vi "ziSaveSettings.vi"(3 "Error In":errorcluster, 4 "Path (\"\")":string, 5 "file path (dialog if empty)":path, 6 "Handle In":T1 {"Handle" format="0x%08x"; "Conn" format="0x%08x"}) -> (0 "Error Out":errorcluster, 1 "Saved Array":string[][](array[string]), 2 "Handle Out":T1 {"Handle" format="0x%08x"; "Conn" format="0x%08x"})   [LabVIEW 2015, in "Zurich Instruments LabOne.lvlib"]
uses:
  Zurich Instruments LabOne.lvlib
  <vilib>/Utility/file.llb/Write To Spreadsheet File (string).vi
  <vilib>/regexp/Match Regular Expression.xnode
  ziTypeHandle.ctl
panel:
  out "node_paths":string[](array[string])
  out "node_values":string[](array[string])
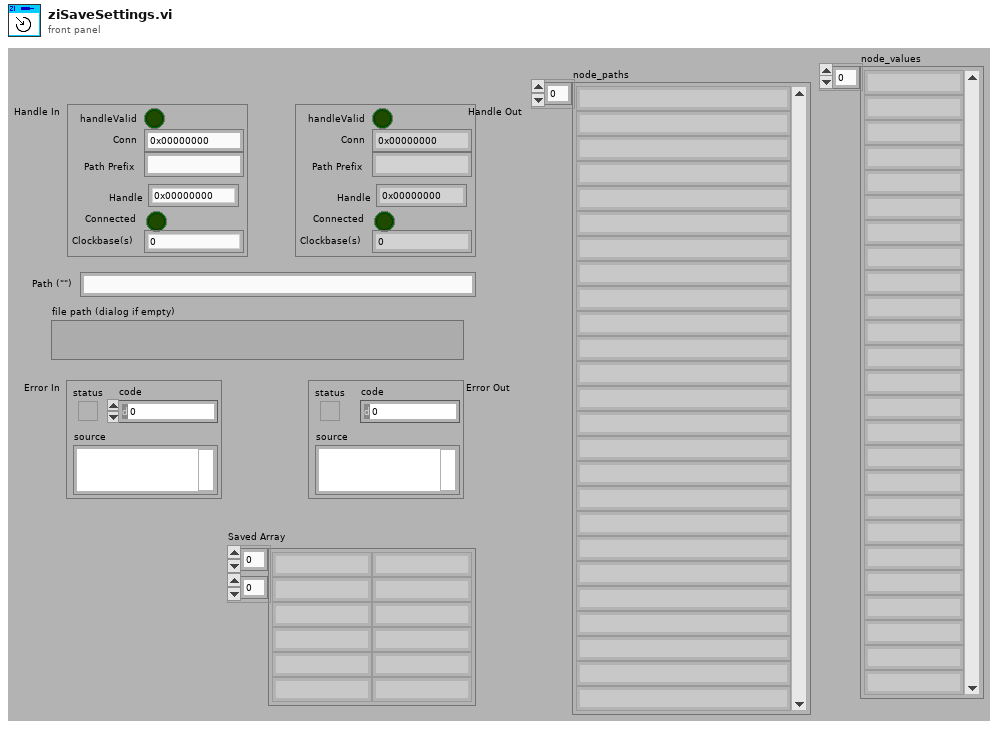
[diagram p1: front panel]
types:
  T1 = typedef "Zurich Instruments LabOne.lvlib/ziTypeHandle.ctl" = cluster{"handleValid":bool, "Conn":u64, "Path Prefix":string, "Handle":u64, "Connected":bool, "Clockbase(s)":dbl}
  T2 = cluster{"Recursive":bool, "Absolut":bool, "Leafs Only":bool, "Settings Only":bool}
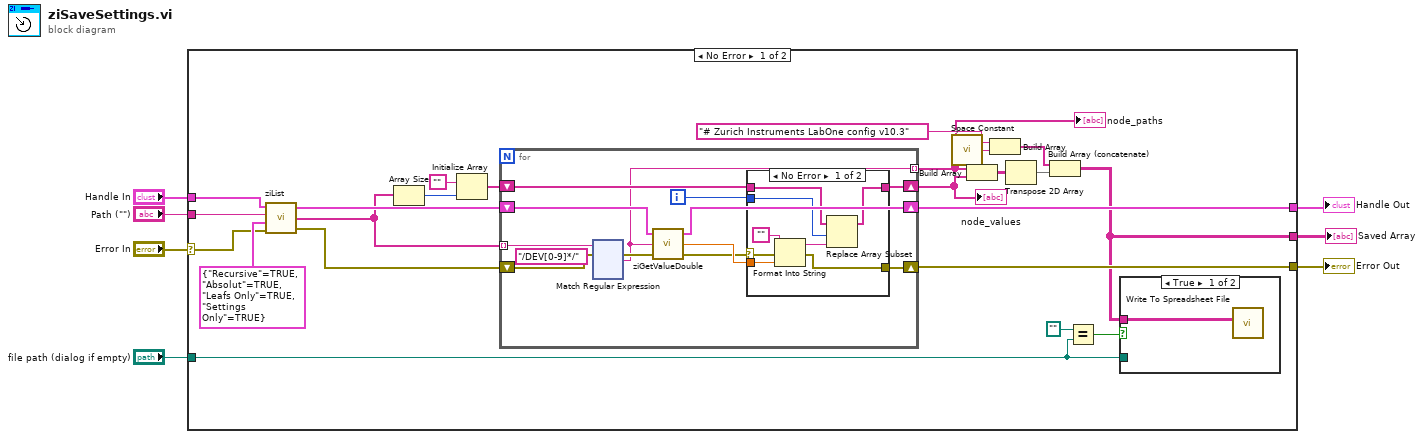
[diagram p0: block diagram]
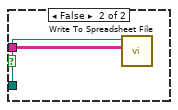
[diagram p2: hidden frame]
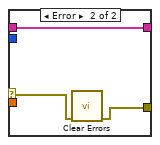
[diagram p3: hidden frame]
diagram:
  n1 = case shown="No Error" "Error In" {
    selector: "Error In" -> [w8 w164]
    tunnel: [w28 w165] -> w7
    tunnel: [w27 w164] -> w6
    tunnel: "file path (dialog if empty)" -> [w11 _]
    tunnel: "Handle In" -> [w25 w165]
    tunnel: "Path (\"\")" -> [w24 _]
    tunnel: [w15 _] -> w2
    frame No Error {
      n2 = call "ziList.vi"("Error In"=w8, "Flags (None)"=T2 {"Recursive"=TRUE, "Absolut"=TRUE, "Leafs Only"=TRUE, "Settings Only"=TRUE}, "Path (\"\")"=w24, "Handle In"=w25) -> ("Error Out"=w29:errorcluster, "Nodes"=w13:string[], "Handle Out"=w30:T1)
      n3 = Array Size(array=w13) -> (size(s)=w20:i32)
      n4 = Initialize Array("", w20) -> (w19:string[])
      n5 = for {
        shift-right: [w41] -> w27
        shift-left: w29 -> [w44]
        shift-right: [w43] -> w28
        shift-left: w30 -> [w45]
        tunnel: w13 -> [w37] mode=indexing
        shift-right: [w39] -> w26
        shift-left: w19 -> [w40]
        tunnel: [w35] -> w12 mode=indexing
        i -> [w38]
        n6 = xnode "Match Regular Expression"("input string"=w37, "regular expression"="/DEV[0-9]*/") -> ("after match"=w35:string)  [unwired: 4 in, 4 out]
        n7 = call "ziGetValueDouble.vi"("error in"=w44, "Path"=w35, "Handle in"=w45) -> ("error out"=w34:errorcluster, "Value"=w42:dbl, "Handle out"=w43:T1)
        n8 = case shown="No Error" w34 {
          selector: w34 -> [w46 w54]
          tunnel: w42 -> [w53 _]
          tunnel: [w52 w55] -> w41
          tunnel: w40 -> [w50 w56]
          tunnel: [w49 w56] -> w39
          tunnel: w38 -> [w47 _]
          frame No Error {
            n9 = Format Into String(initial string="", error in=w46, w53) -> (resulting string=w51:string, error out=w52:errorcluster)  [unwired: 1 in]
            n10 = Replace Array Subset(array=w50, new element=w51, index=w47) -> (w49:string[])
          }
          frame Error {
            n11 = call <vilib>:"Clear Errors.vi"("error in (no error)"=w54) -> ("error out"=w55:errorcluster)  [unwired: 5 in, 1 out]
          }
        }
      }
      "node_values" <- w26
      "node_paths" <- w12
      n12 = call <vilib>:"Space Constant.vi"() -> ("String"=w21:string)
      n13 = Build Array(w12, w26) -> (w18:string[][])
      n14 = Build Array("# Zurich Instruments LabOne config v10.3" ("new element/subarray"), w21) -> (w17:string[])
      n15 = Transpose 2D Array(2D array=w18) -> (transposed array=w16:string[][])
      n16 = Build Array (concatenate)(w17, w16) -> (w15:string[][])
      n17 = Equal?(x=path "", y=w11) -> (x = y?=w10:bool)
      n18 = case shown="True" w10 {
        tunnel: w15 -> [w31 w33]
        tunnel: w11 -> [_ w32]
        frame True {
          n19 = call-poly <vilib>:"Write To Spreadsheet File.vi"("2D data"=w31) -> ()  [unwired: 7 in, 1 out]
        }
        frame False {
          n20 = call-poly <vilib>:"Write To Spreadsheet File.vi"("2D data"=w33, "file path (dialog if empty)"=w32) -> ()  [unwired: 6 in, 1 out]
        }
      }
    }
    frame Error {
    }
  }
  "Handle Out" <- w7
  "Error Out" <- w6
  "Saved Array" <- w2
